vi "Convert Channel Tag And Name.vi"(7 "Direction":enum16{"Tag to Name", "Name to Tag"}(ring), 10 "String[] in":string[](array[string])) -> (2 "String[] out":string[](array[string]), 3 "Unit[]":string[](array[string]))   [LabVIEW 2016]
uses:
  DAQ-Config/SubVIs/FGV_Cards.ctl
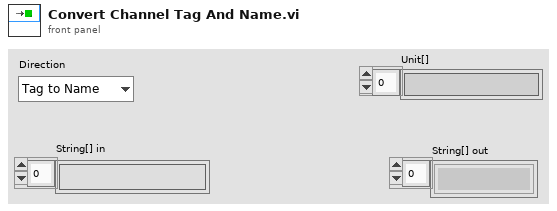
[diagram p1: front panel]
types:
  T1 = typedef "FGV_Cards.ctl" = enum16{"Initlize", "Set_DAQCards", "Set_VCHCards", "Get_DAQCards", "Get_VCHCards", "Get_ALLUsing"}
  T2 = typedef "PSCHN_Card Para.ctl" = cluster{"Module Type":string, "Module Name":string, "ModuSN":string, "ModuIP":string, "Used?":bool, "Connected":bool, "Timing*":cluster{"Sample Rate":dbl}, "Channels":T3[]}
  T3 = typedef "PSCHN_Channel Para.ctl" = cluster{"CHTag*":string, "Used?*":bool, "CHName":string, "Unit":string, "斜率":dbl, "截距":dbl}
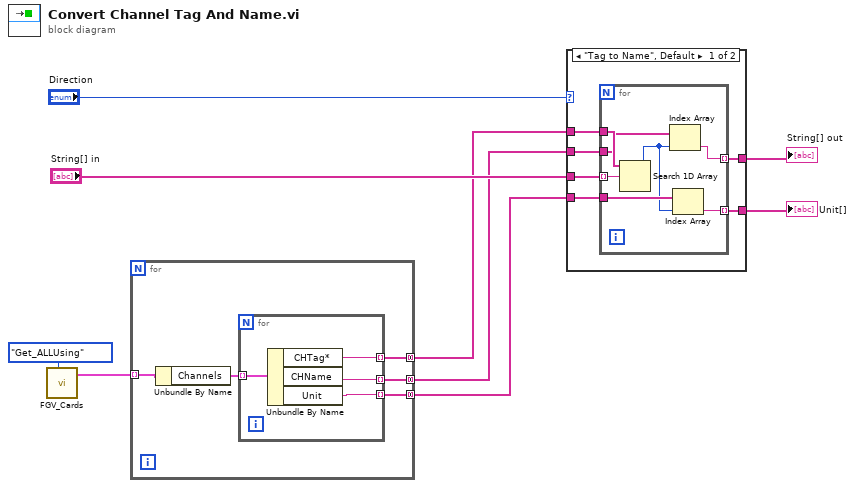
[diagram p0: block diagram]
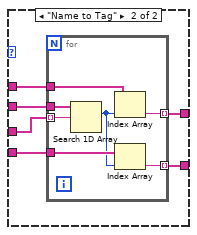
[diagram p2: hidden frame]
diagram:
  n1 = call "FGV_Cards.vi"("Action"=FGV_Cards."Get_ALLUsing") -> ("Cards out"=w4:T2[])  [unwired: 9 in, 1 out]
  n2 = for {
    tunnel: w4 -> [w14] mode=indexing
    tunnel: [w12] -> w6 mode=concatenating
    tunnel: [w11] -> w5 mode=concatenating
    tunnel: [w10] -> w2 mode=concatenating
    n3 = Unbundle By Name(w14) -> ("Channels"=w13:T3[])
    n4 = for {
      tunnel: w13 -> [w18] mode=indexing
      tunnel: [w17] -> w12 mode=indexing
      tunnel: [w16] -> w11 mode=indexing
      tunnel: [w15] -> w10 mode=indexing
      n5 = Unbundle By Name(w18) -> ("CHTag*"=w17:string, "CHName"=w16:string, "Unit"=w15:string)
    }
  }
  n6 = case shown="\"Tag to Name\", Default" "Direction" {
    tunnel: w5 -> [w22 w37]
    tunnel: w6 -> [w24 w36]
    tunnel: "String[] in" -> [w23 w35]
    tunnel: [w21 w34] -> w9
    tunnel: w2 -> [w20 w33]
    tunnel: [w19 w32] -> w1
    frame "Tag to Name", Default {
      n7 = for {
        tunnel: w24 -> [w31]
        tunnel: w23 -> [w30] mode=indexing
        tunnel: w22 -> [w29]
        tunnel: [w28] -> w21 mode=indexing
        tunnel: w20 -> [w27]
        tunnel: [w25] -> w19 mode=indexing
        n8 = Search 1D Array(1D array=w31, element=w30) -> (index of element=w26:i32)  [unwired: 1 in]
        n9 = Index Array(array=w29, index=w26) -> (element=w28:string)
        n10 = Index Array(array=w27, index=w26) -> (element=w25:string)
      }
    }
    frame "Name to Tag" {
      n11 = for {
        tunnel: w37 -> [w44]
        tunnel: w36 -> [w43]
        tunnel: w35 -> [w42] mode=indexing
        tunnel: [w41] -> w34 mode=indexing
        tunnel: w33 -> [w40]
        tunnel: [w38] -> w32 mode=indexing
        n12 = Search 1D Array(1D array=w44, element=w42) -> (index of element=w39:i32)  [unwired: 1 in]
        n13 = Index Array(array=w43, index=w39) -> (element=w41:string)
        n14 = Index Array(array=w40, index=w39) -> (element=w38:string)
      }
    }
  }
  "String[] out" <- w9
  "Unit[]" <- w1
